vi "File.Rotate.Manager.vi"(9 "Q Name":string="FileRotate", 11 "Config Folder":path) -> ()   [LabVIEW 2018]
uses:
  <vilib>/KATE/Queues/Queue Utils.lvlib
  <vilib>/KATE/Files/File Utils.lvlib
  <vilib>/KATE/Scheduler/Scheduler.lvlib
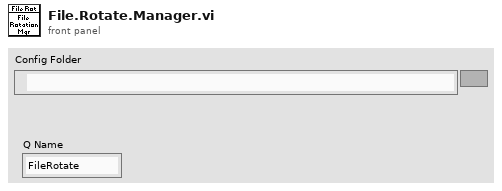
[diagram p1: front panel]
types:
  T1 = cluster{"Folder":path, "Max SubDirs":i32, "Max Files":i32, "Interval(Days)":dbl, "LastCheck(s)":dbl}
  T2 = cluster{"Folder":path, "Max SubDirs":i32, "Max Files":i32, "Interval(Days)":dbl, "LastCheck(s)":dbl}[]
  T3 = cluster{"Config Folder":path, "Tasks":cluster{"Folder":path, "Max SubDirs":i32, "Max Files":i32, "Interval(Days)":dbl, "LastCheck(s)":dbl}[]}
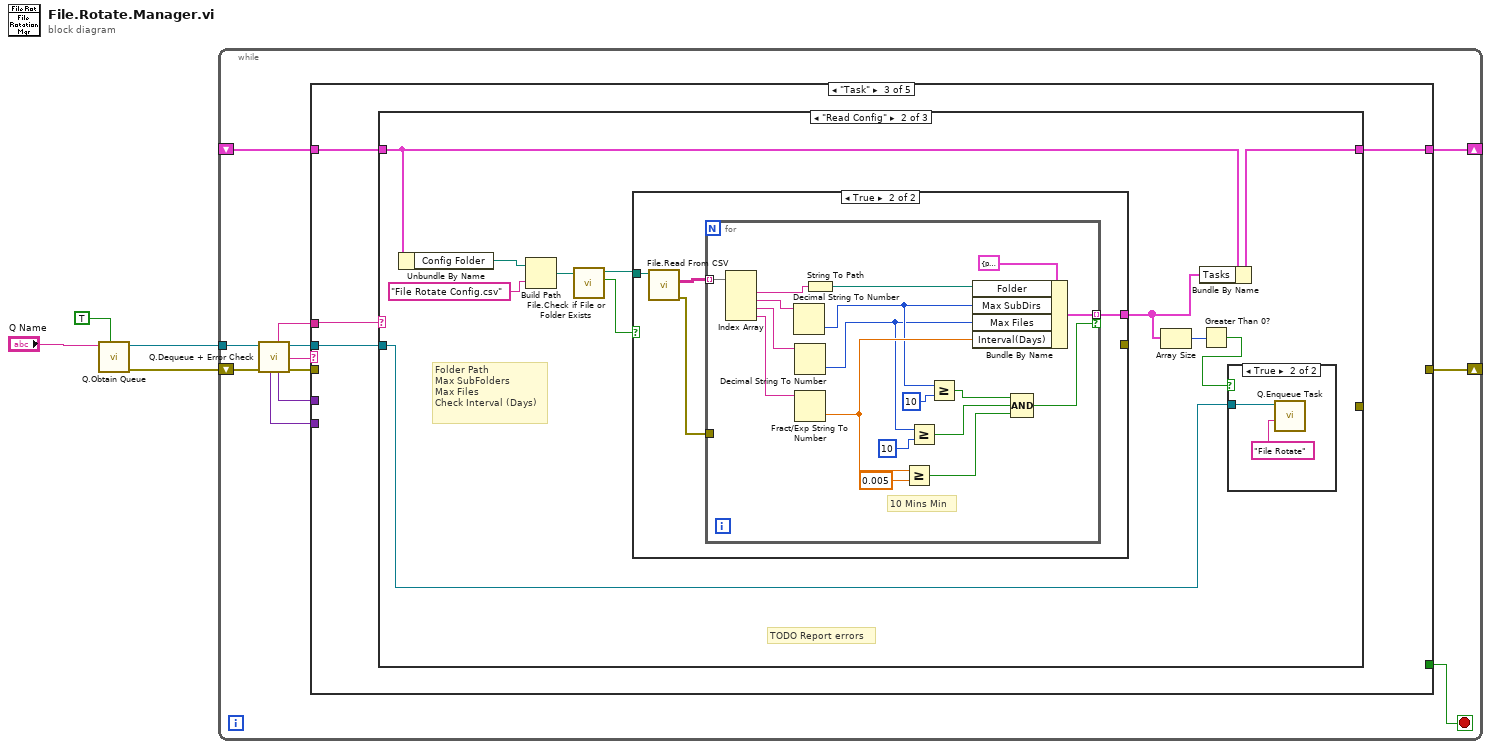
[diagram p0: block diagram]
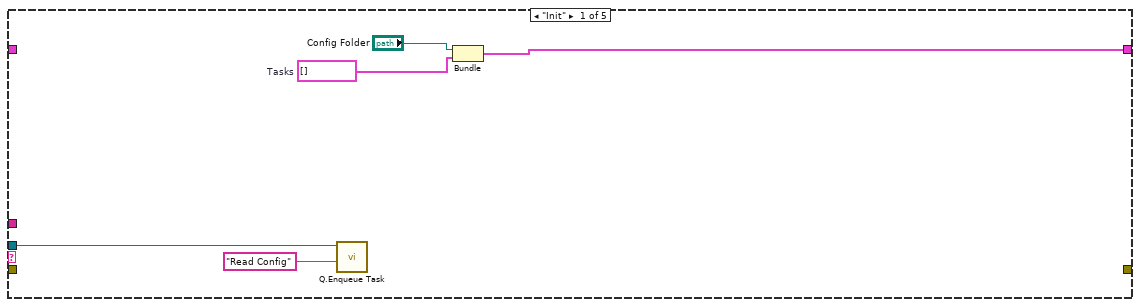
[diagram p2: hidden frame]
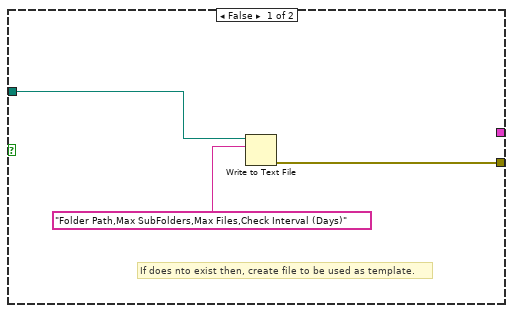
[diagram p6: hidden frame]
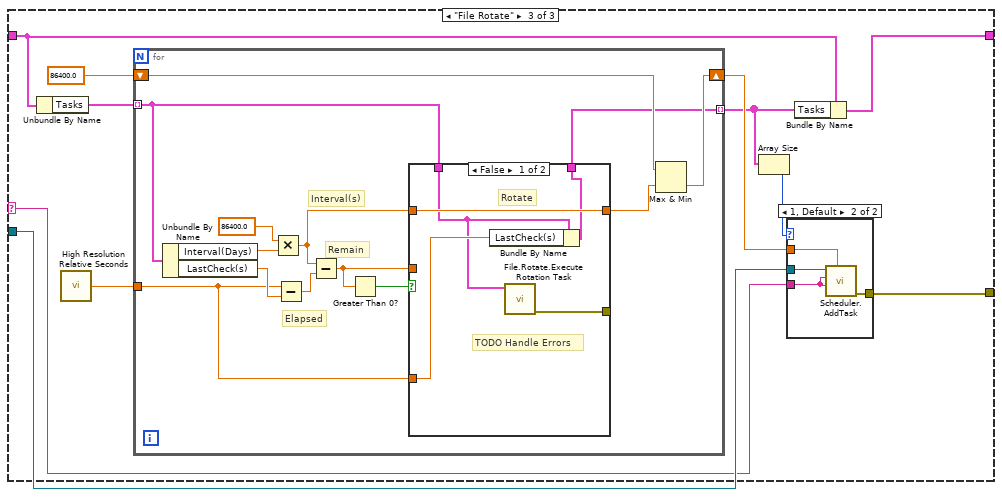
[diagram p7: hidden frame]
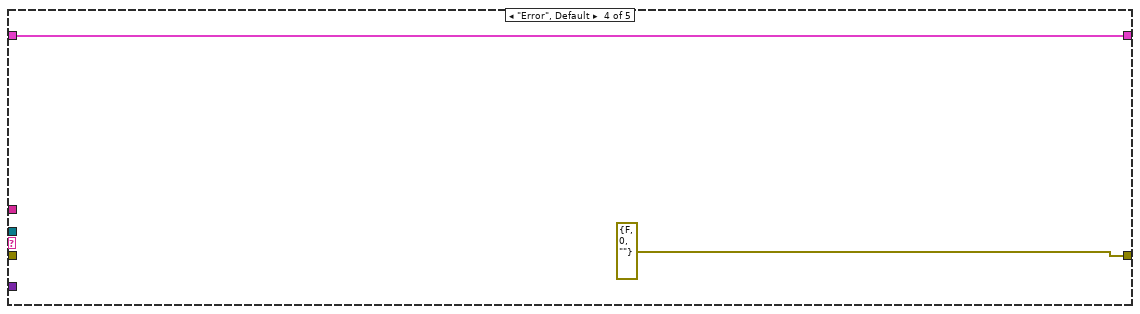
[diagram p10: hidden frame]
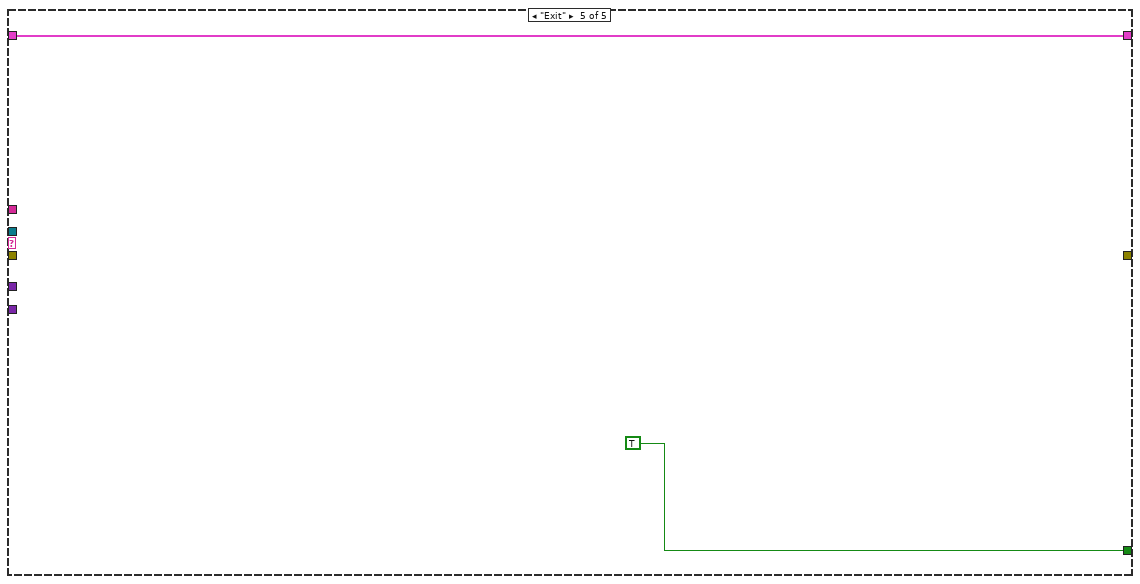
[diagram p11: hidden frame]
diagram:
  n1 = call <vilib>:"Q.Obtain Queue.vi"("Enqueue Init"=TRUE, "Q Name"="Q Name") -> ("error out"=w4:errorcluster, "Q Out"=w1:refnum<queue>)  [unwired: 7 in, 1 out]
  n2 = while {
    shift-right: [w7] -> _
    shift-left: w4 -> [w16]
    tunnel: w1 -> [w9]
    shift-right: [w5] -> _
    shift-left: _ -> [w6]
    stop <- w8 stop-if-true
    n3 = call <vilib>:"Q.Dequeue + Error Check.vi"("Error In"=w16, "Q In"=w9) -> ("error out"=w15:errorcluster, "Cmd"=w14:string, "Q Out"=w13:refnum<queue>, "Data1"=w11:variant, "Sub"=w12:string, "Data2"=w10:variant)  [unwired: 4 in]
    n4 = case shown="\"Task\"" w14 {
      tunnel: w15 -> [_ _ _ _ _]
      tunnel: w13 -> [w18 _ w23 _ _]
      tunnel: w12 -> [_ _ w26 _ _]
      tunnel: w11 -> [_ _ _ _ _]
      tunnel: w10 -> [_ _ _ _ _]
      tunnel: [_ _ _ _ TRUE] -> w8
      tunnel: [_ _ _ errorcluster {"status"=FALSE, "code"=0, "source"=""} ("error constant") _] -> w7
      tunnel: w6 -> [_ w22 w25 w101 w103]
      tunnel: [w19 w22 w24 w101 w103] -> w5
      frame "Init" {
        w20 = T2 []  # Tasks
        n5 = call <vilib>:"Q.Enqueue Task.vi"("Task Name"="Read Config", "Q In"=w18) -> ()  [unwired: 8 in, 2 out]
        n6 = Bundle("Config Folder"="Config Folder", "Tasks"=w20) -> (w19:T3)  [unwired: 1 in]
      }
      frame "Reset" {
      }
      frame "Task" {
        n7 = case shown="\"Read Config\"" w26 {
          selector: w26 -> [_ _ w68]
          tunnel: w25 -> [w27 w35 w75]
          tunnel: [w27 w36 w76] -> w24
          tunnel: w23 -> [_ w32 w72]
          tunnel: [_ _ w69] -> _
          frame Default {
          }
          frame "Read Config" {
            # "TODO Report errors"
            # "Folder Path\nMax SubFolders\nMax Files\nCheck Interval (Days)"
            n8 = Unbundle By Name(w35) -> ("Config Folder"=w38:path)
            n9 = Build Path(base path=w38, name or relative path="File Rotate Config.csv") -> (appended path=w30:path)
            n10 = call <vilib>:"File.Check if File or Folder Exists.vi"("Path"=w30) -> ("Exists"=w28:bool, "Dup Path"=w29:path)  [unwired: 6 in, 3 out]
            n11 = case shown="True" w28 {
              tunnel: w29 -> [w43 w47]
              tunnel: [_ w45] -> w34
              tunnel: [w41 _] -> _
              frame False {
                # "If does nto exist then, create file to be used as template."
                n12 = Write to Text File(file (use dialog)=w43, text="Folder Path,Max SubFolders,Max Files,Check Interval (Days)") -> (error out=w41:errorcluster)  [unwired: 2 in, 2 out]
              }
              frame True {
                n13 = call <vilib>:"File.Read From CSV.vi"("File"=w47) -> ("error out"=w44:errorcluster, "Data"=w46:string[][])  [unwired: 8 in, 1 out]
                n14 = for {
                  tunnel: w46 -> [w65] mode=indexing
                  tunnel: [w63] -> w45 mode=indexing if=w48
                  tunnel: w44 -> [_]
                  # "10 Mins Min"
                  n15 = Index Array(array=w65) -> (element #1=w62:string, element #2=w61:string, element #3=w60:string, element #4=w59:string)  [unwired: 4 in]
                  n16 = Decimal String To Number(string=w61) -> (number=w55:i32)  [unwired: 2 in, 1 out]
                  n17 = Decimal String To Number(string=w60) -> (number=w54:i32)  [unwired: 2 in, 1 out]
                  n18 = Fract/Exp String To Number(string=w59) -> (number=w57:dbl)  [unwired: 3 in, 1 out]
                  n19 = String To Path(string=w62) -> (path=w58:path)
                  n20 = Greater Or Equal?(x=w57, y=0.005) -> (x >= y?=w49:bool)
                  n21 = Greater Or Equal?(x=w54, y=10) -> (x >= y?=w50:bool)
                  n22 = Greater Or Equal?(x=w55, y=10) -> (x >= y?=w51:bool)
                  n23 = Bundle By Name(cluster=T1 {"Folder"=path "", "Max SubDirs"=0, "Max Files"=0, "Interval(Days)"=0.0, "LastCheck(s)"=0.0}, "Folder"=w58, "Max SubDirs"=w55, "Max Files"=w54, "Interval(Days)"=w57) -> (w63:T1)
                  n24 = Compound Arithmetic op=AND(w51, w50, w49) -> (w48:bool)
                }
              }
            }
            n25 = Array Size(array=w34) -> (size(s)=w33:i32)
            n26 = Bundle By Name(cluster=w35, "Tasks"=w34) -> (w36:T3)
            n27 = Greater Than 0?(x=w33) -> (x > 0?=w31:bool)
            n28 = case shown="True" w31 {
              tunnel: w32 -> [_ w39]
              frame False {
              }
              frame True {
                n29 = call <vilib>:"Q.Enqueue Task.vi"("Task Name"="File Rotate", "Q In"=w39) -> ()  [unwired: 8 in, 2 out]
              }
            }
          }
          frame "File Rotate" {
            n30 = Unbundle By Name(w75) -> ("Tasks"=w74:T2)
            n31 = call <vilib>:"High Resolution Relative Seconds.vi"() -> ("relative seconds"=w73:dbl)
            n32 = for {
              tunnel: w74 -> [w82] mode=indexing
              tunnel: w73 -> [w81]
              shift-right: [w87] -> w70
              shift-left: 86400.0 -> [w86]
              tunnel: [w83] -> w67 mode=indexing
              # "Interval(s)"
              # "Elapsed"
              # "Remain"
              n33 = Unbundle By Name(w82) -> ("Interval(Days)"=w92:dbl, "LastCheck(s)"=w93:dbl)
              n34 = Multiply(x=86400.0 ("y"), y=w92) -> (x*y=w85:dbl)
              n35 = Subtract(x=w81, y=w93) -> (x-y=w90:dbl)
              n36 = Subtract(x=w85, y=w90) -> (x-y=w88:dbl)
              n37 = Greater Than 0?(x=w88) -> (x > 0?=w89:bool)
              n38 = case shown="False" w89 {
                tunnel: w88 -> [_ w100]
                tunnel: w85 -> [w98 _]
                tunnel: [w98 w100] -> w84
                tunnel: [w97 w99] -> w83
                tunnel: w82 -> [w95 w99]
                tunnel: w81 -> [w96 _]
                tunnel: [w94 _] -> _
                frame False {
                  # "TODO Handle Errors"
                  # "Rotate"
                  n39 = Bundle By Name(cluster=w95, "LastCheck(s)"=w96) -> (w97:T1)
                  n40 = call "File.Rotate.Execute Rotation Task.vi"("Task"=w95) -> ("error out"=w94:errorcluster)  [unwired: 10 in]
                }
                frame True {
                }
              }
              n41 = Max & Min(x=w86, y=w84) -> (min(x,y)=w87:dbl)  [unwired: 1 out]
            }
            n42 = Array Size(array=w67) -> (size(s)=w66:i32)
            n43 = case shown="1, Default" w66 {
              tunnel: w72 -> [_ w80]
              tunnel: w70 -> [_ w79]
              tunnel: [_ w78] -> w69
              tunnel: w68 -> [_ w77]
              frame 0 {
              }
              frame 1, Default {
                n44 = call <vilib>:"Scheduler.AddTask.vi"("Interval(s)"=w79, "Task Name"=w77, "Sched Name"=w77, "Q In"=w80) -> ("Error Out"=w78:errorcluster)  [unwired: 6 in, 1 out]
              }
            }
            n45 = Bundle By Name(cluster=w75, "Tasks"=w67) -> (w76:T3)
          }
        }
      }
      frame "Error", Default {
      }
      frame "Exit" {
      }
    }
  }
